vi "Windspeed Warnings.vi"(10 "최고 풍속":dbl, 11 "현재 풍속":dbl) -> (2 "풍속 경고 텍스트":string="경고 없음", 3 "풍속 경고?":bool)   [LabVIEW 2014]
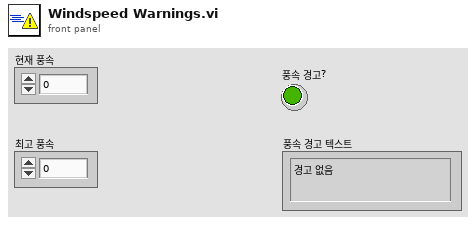
[diagram p1: front panel]
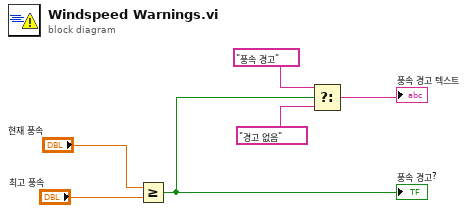
[diagram p0: block diagram]
diagram:
  n1 = Greater Or Equal?(x="현재 풍속", y="최고 풍속") -> (x >= y?=w4:bool)
  "풍속 경고?" <- w4
  n2 = Select(t="풍속 경고", s=w4, f="경고 없음") -> (s? t:f=→"풍속 경고 텍스트":string)
